vi "write_tag_status_2.vi"(9 "Inicio pasada 3":timestamp=timestamp(3789638435.424 s since 1904-01-01), 10 "Train":string[](array[string]), 11 "file path (use dialog)":path=path "c:/RFID/status.csv") -> ()   [LabVIEW 2015]
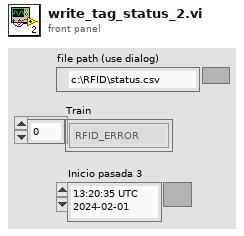
[diagram p1: front panel]
types:
  T1 = enum16{"open", "replace", "create", "open or create", "replace or create", "replace or create with confirmation"}
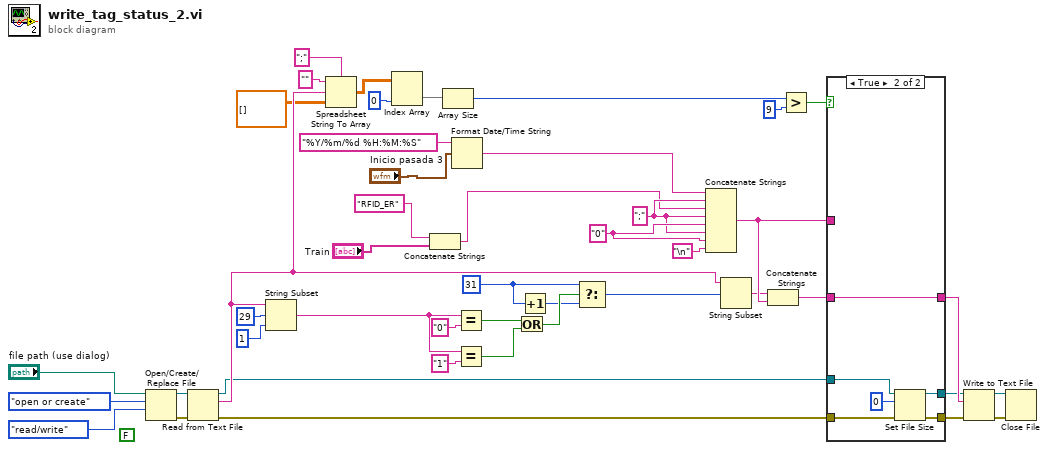
[diagram p0: block diagram]
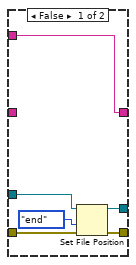
[diagram p2: hidden frame]
diagram:
  w45 = "0" ("string")
  w37 = 31 ("offset (0)")
  w35 = ";" ("string")
  (unwired) FALSE ("disable buffering (F)")
  n1 = Open/Create/Replace File(file path (use dialog)="file path (use dialog)", operation (0:open)=T1."open or create", access (0:read/write)=enum16{"read/write", "read-only", "write-only"}."read/write") -> (refnum out=w12:refnum<file>, error out=w13:errorcluster)  [unwired: 2 in, 2 out]
  n2 = Read from Text File(file (use dialog)=w12, error in=w13) -> (refnum out=w14:refnum<file>, text=w29:string, error out=w15:errorcluster)  [unwired: 2 in, 1 out]
  n3 = String Subset(string=w29, offset (0)=29, length (rest)=1 ("length (rest)")) -> (substring=w42:string)
  n4 = Spreadsheet String To Array(delimiter (Tab)=";", format string="", spreadsheet string=w29, array type (2D Dbl)=dbl[][] []) -> (array=w19:dbl[][])
  n5 = Index Array(array=w19, index (col)=0 ("index (row)")) -> (element=w20:dbl[])  [unwired: 1 in]
  n6 = Concatenate Strings("RFID_ER" ("Train"), "Train") -> (w3:string)
  n7 = Array Size(array=w20) -> (size(s)=w22:i32)
  n8 = Format Date/Time String(time format string (%c)="%Y/%m/%d %H:%M:%S", seconds (now)="Inicio pasada 3") -> (date/time string=w7:string)  [unwired: 1 in]
  n9 = Equal?(x=w42, y="0") -> (x = y?=w39:bool)
  n10 = Equal?(x=w42, y="1") -> (x = y?=w40:bool)
  n11 = Or(x=w39, y=w40) -> (x .or. y?=w38:bool)
  n12 = Increment(x=w37) -> (x+1=w26:i32)
  n13 = Select(t=w37, s=w38, f=w26) -> (s? t:f=w27:i32)
  n14 = Concatenate Strings(w7, w35, w3, w35, w45, w35, w45, "\n") -> (w33:string)
  n15 = String Subset(string=w29, offset (0)=w27) -> (substring=w30:string)  [unwired: 1 in]
  n16 = Concatenate Strings(w30, w33) -> (w32:string)
  n17 = Greater?(x=w22, y=9) -> (0:w31:bool)
  n18 = case shown="True" w31 {
    tunnel: [w50 w54] -> w10
    tunnel: [w49 w55] -> w11
    tunnel: w14 -> [w48 w56]
    tunnel: w15 -> [w47 w53]
    tunnel: [w46 w57] -> w34
    tunnel: w32 -> [_ w57]
    tunnel: w33 -> [w46 _]
    frame False {
      n19 = Set File Position(refnum=w48, from (0:start)=enum16{"start", "end", "current"}."end", error in=w47) -> (refnum out=w49:refnum<file>, error out=w50:errorcluster)  [unwired: 1 in]
    }
    frame True {
      n20 = Set File Size(4:w53, 6:i64 0 ("size (in bytes)"), 7:w56) -> (0:w54:errorcluster, 3:w55:refnum<file>)
    }
  }
  n21 = Write to Text File(file (use dialog)=w11, text=w34, error in=w10) -> (refnum out=w8:refnum<file>, error out=w9:errorcluster)  [unwired: 1 in, 1 out]
  n22 = Close File(refnum=w8, error in=w9) -> ()  [unwired: 2 out]
